vi "Eurotherm_write_H.vi"(8 "error in (no error)":errorcluster, 9 "HR_sp":dbl min=0.0 max=100.0 step=0.1, 10 "HR write":bool, 11 "Modbus Master in":refnum<class "Modbus Master.lvclass">) -> (0 "error out":errorcluster, 3 "Modbus Master out":refnum<class "Modbus Master.lvclass">)   [LabVIEW 2022 SP3, in "CC_Library.lvlib"]
uses:
  CC_Library.lvlib
  <vilib>/Modbus/master/Modbus Master.lvclass
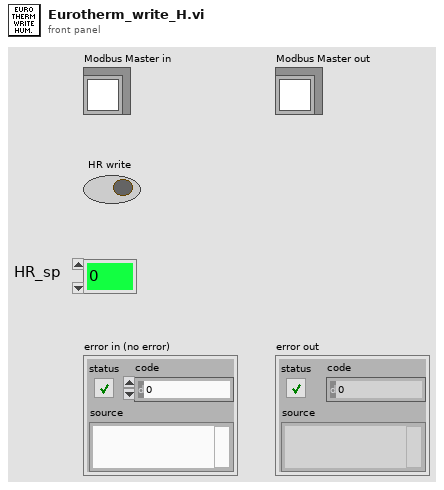
[diagram p1: front panel]
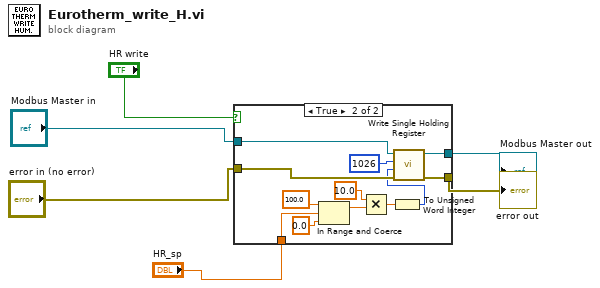
[diagram p0: block diagram]
diagram:
  n1 = case shown="True" "HR write" {
    tunnel: "error in (no error)" -> [w7 w20]
    tunnel: "Modbus Master in" -> [w8 w18]
    tunnel: [w7 w17] -> w4
    tunnel: [w8 w16] -> w3
    tunnel: "HR_sp" -> [_ w9]
    frame False {
    }
    frame True {
      n2 = In Range and Coerce(upper limit=100.0, x=w9, lower limit=0.0) -> (coerced(x)=w11:dbl)  [unwired: 1 out]
      n3 = Multiply(x=10.0, y=w11) -> (x*y=w10:dbl)
      n4 = To Unsigned Word Integer(number=w10) -> (unsigned 16bit integer=w15:u16)
      n5 = call-dynamic "Write Single Holding Register.vi"("error in (no error)"=w20, "holding register value"=w15, "address"=u16 1026, "Modbus master in"=w18) -> ("error out"=w17:errorcluster, "Modbus master out"=w16:refnum<class "Modbus Master.lvclass">)  [unwired: 6 in]
    }
  }
  "error out" <- w4
  "Modbus Master out" <- w3
